vi "origin.vi"(1 "origin":T1) -> (0 "urdf out":string)   [LabVIEW 2010]
uses:
  Position.ctl
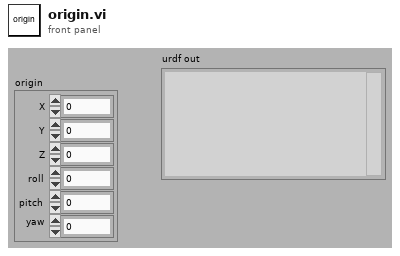
[diagram p1: front panel]
types:
  T1 = typedef "Position.ctl" = cluster{"X":sgl, "Y":sgl, "Z":sgl, "roll":sgl, "pitch":sgl, "yaw":sgl}
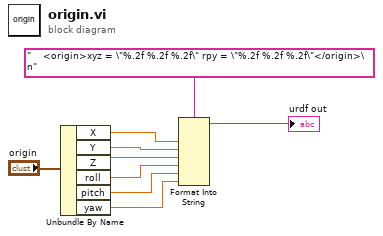
[diagram p0: block diagram]
diagram:
  n1 = Unbundle By Name("origin") -> ("X"=w6:sgl, "Y"=w5:sgl, "Z"=w4:sgl, "roll"=w3:sgl, "pitch"=w2:sgl, "yaw"=w1:sgl)
  n2 = Format Into String(format string="    <origin>xyz = \"%.2f %.2f %.2f\" rpy = \"%.2f %.2f %.2f\"</origin>\n", w6, w5, w4, w3, w2, w1) -> (resulting string=→"urdf out":string)  [unwired: 2 in, 1 out]
